vi "SCD - Write Engineering Data to File.vi"(8 "error in":errorcluster, 9 "Temp Data":dbl[](array[numeric]), 10 "mesage":string, 11 "Base SCD Log File Folder (User must create)":path=path "C:/SCMP Logs") -> (0 "error out":errorcluster, 2 "Recent Log":string="\r", 3 "first call":bool, 5 "Today's SCD Engineering File":path)   [LabVIEW 2014]
doc: "This vi create or open file, which is save in format YYYYMMDD.txt. In this file are logs from CoMP-S Main program."
panel:
  out "spreadsheet string":string
  out "date/time string":string
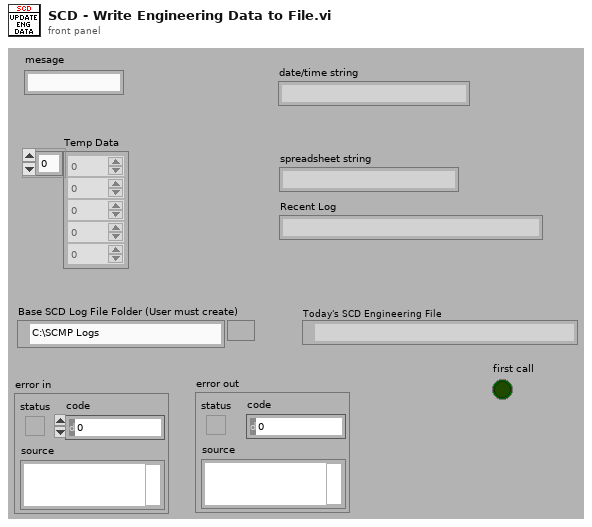
[diagram p1: front panel]
types:
  T1 = enum16{"open", "replace", "create", "open or create", "replace or create", "replace or create with confirmation"}
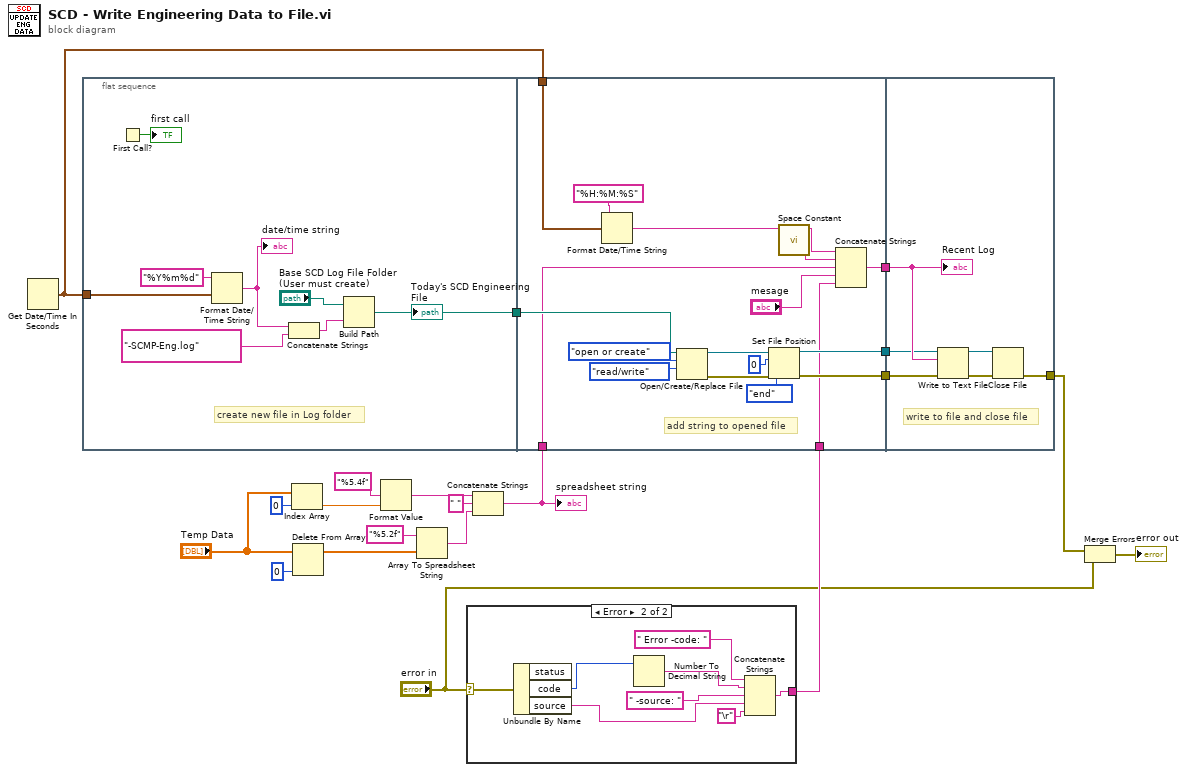
[diagram p0: block diagram]
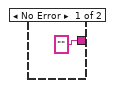
[diagram p2: hidden frame]
diagram:
  n1 = Get Date/Time In Seconds() -> (seconds since 1Jan1904=w20:timestamp)
  n2 = flat-sequence {
    tunnel: w20 -> [w26]
    tunnel: [w22] -> w19
    tunnel: w20 -> [w41]
    tunnel: w19 -> [w40]
    tunnel: [w39] -> w18
    tunnel: [w33] -> w17
    tunnel: w10 -> [w37]
    tunnel: [w34] -> w15
    tunnel: w12 -> [w30]
    tunnel: w18 -> [w49]
    tunnel: w17 -> [w48]
    tunnel: w15 -> [w47]
    tunnel: [w46] -> w13
    frame #0 {
      # "create new file in Log folder"
      n3 = First Call?() -> (First Call?: T/F=→"first call":bool)
      n4 = Format Date/Time String(time format string (%c)="%Y%m%d", seconds (now)=w26) -> (date/time string=w25:string)  [unwired: 1 in]
      "date/time string" <- w25
      n5 = Concatenate Strings(w25, "-SCMP-Eng.log" ("string")) -> (w24:string)
      n6 = Build Path(base path="Base SCD Log File Folder (User must create)", name or relative path=w24) -> (appended path=w22:path)
      "Today's SCD Engineering File" <- w22
    }
    frame #1 {
      # "add string to opened file"
      n7 = Format Date/Time String(time format string (%c)="%H:%M:%S", seconds (now)=w41) -> (date/time string=w43:string)  [unwired: 1 in]
      n8 = Open/Create/Replace File(file path (use dialog)=w40, operation (0:open)=T1."open or create", access (0:read/write)=enum16{"read/write", "read-only", "write-only"}."read/write") -> (refnum out=w35:refnum<file>, error out=w36:errorcluster)  [unwired: 1 in, 3 out]
      n9 = Set File Position(offset (in bytes) (0)=i64 0, refnum=w35, from (0:start)=enum16{"start", "end", "current"}."end", error in=w36) -> (refnum out=w33:refnum<file>, error out=w34:errorcluster)
      n10 = call <vilib>:"Space Constant.vi"() -> ("String"=w42:string)
      n11 = Concatenate Strings(w43, w42, w37, "mesage", w30) -> (w39:string)
    }
    frame #2 {
      # "write to file and close file"
      n12 = Write to Text File(file (use dialog)=w48, text=w49, error in=w47) -> (refnum out=w50:refnum<file>, error out=w51:errorcluster)  [unwired: 1 in, 1 out]
      n13 = Close File(refnum=w50, error in=w51) -> (error out=w46:errorcluster)  [unwired: 1 out]
      "Recent Log" <- w49
    }
  }
  n14 = Index Array(array="Temp Data", index=0) -> (element=w5:dbl)
  n15 = Delete From Array(array="Temp Data", index=0) -> (array with subset deleted=w8:dbl[])  [unwired: 1 in, 1 out]
  n16 = Format Value(format string="%5.4f", value (0)=w5) -> (output string=w3:string)  [unwired: 1 in]
  n17 = Array To Spreadsheet String(array=w8, 3:"%5.2f" ("format string")) -> (spreadsheet string=w2:string)  [unwired: 1 in]
  n18 = case shown="Error" "error in" {
    selector: "error in" -> [_ w57]
    tunnel: ["" w54] -> w12
    frame No Error {
    }
    frame Error {
      n19 = Unbundle By Name(w57) -> ("code"=w56:i32, "source"=w55:string)  [unwired: 1 out]
      n20 = Number To Decimal String(number=w56) -> (decimal integer string=w60:string)  [unwired: 1 in]
      n21 = Concatenate Strings(" Error -code: ", w60, " -source: ", w55, "\r") -> (w54:string)
    }
  }
  n22 = Concatenate Strings(w3, " " ("string"), w2) -> (w10:string)
  "spreadsheet string" <- w10
  n23 = Merge Errors(w13, "error in") -> (→"error out":errorcluster)
